vi "client.vi"() -> ()   [LabVIEW 2019]
uses:
  <vilib>/NI/STM/TCP/Read Meta Data (TCP Ref).vi
  <vilib>/NI/STM/TCP/Get Connection Reference (TCP).vi
  <vilib>/NI/STM/TCP/Read Meta Data (TCP Clst).vi
  <vilib>/NI/STM/TCP/Write Message (TCP).vi
  <vilib>/NI/STM/TCP/Read Message (TCP).vi
  <vilib>/NI/STM/NI STM.lvlib
panel:
  out "MOVE Command":T1
  out "error  out":errorcluster
  in  "stop":bool
  in  "Target IP Address":string="192.168.150.9"
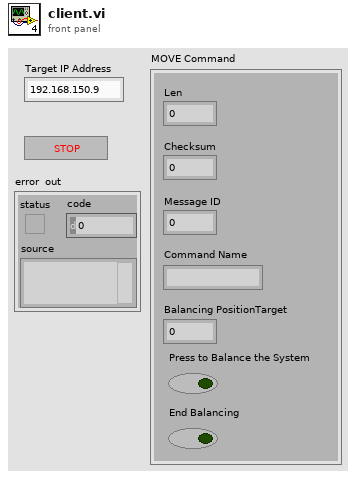
[diagram p1: front panel]
types:
  T1 = cluster{"Len":u8, "Checksum":u16, "Message ID":u16, "Command Name":string, "Balancing PositionTarget ":dbl, "Press to Balance the System":bool, "End Balancing":bool}
  T2 = typedef "NI STM.lvlib/TCP Connection Info.ctl" = cluster{"connection ID":refnum<k5>, "meta data":T3[]}
  T3 = typedef "NI STM.lvlib/MetaDataElement.ctl" = string
  T4 = cluster{"Len":u8, "Checksum":u16, "Message ID":u16, "Command Name":u32, "Balancing PositionTarget ":dbl, "Press to Balance the System":bool, "End Balancing":bool}
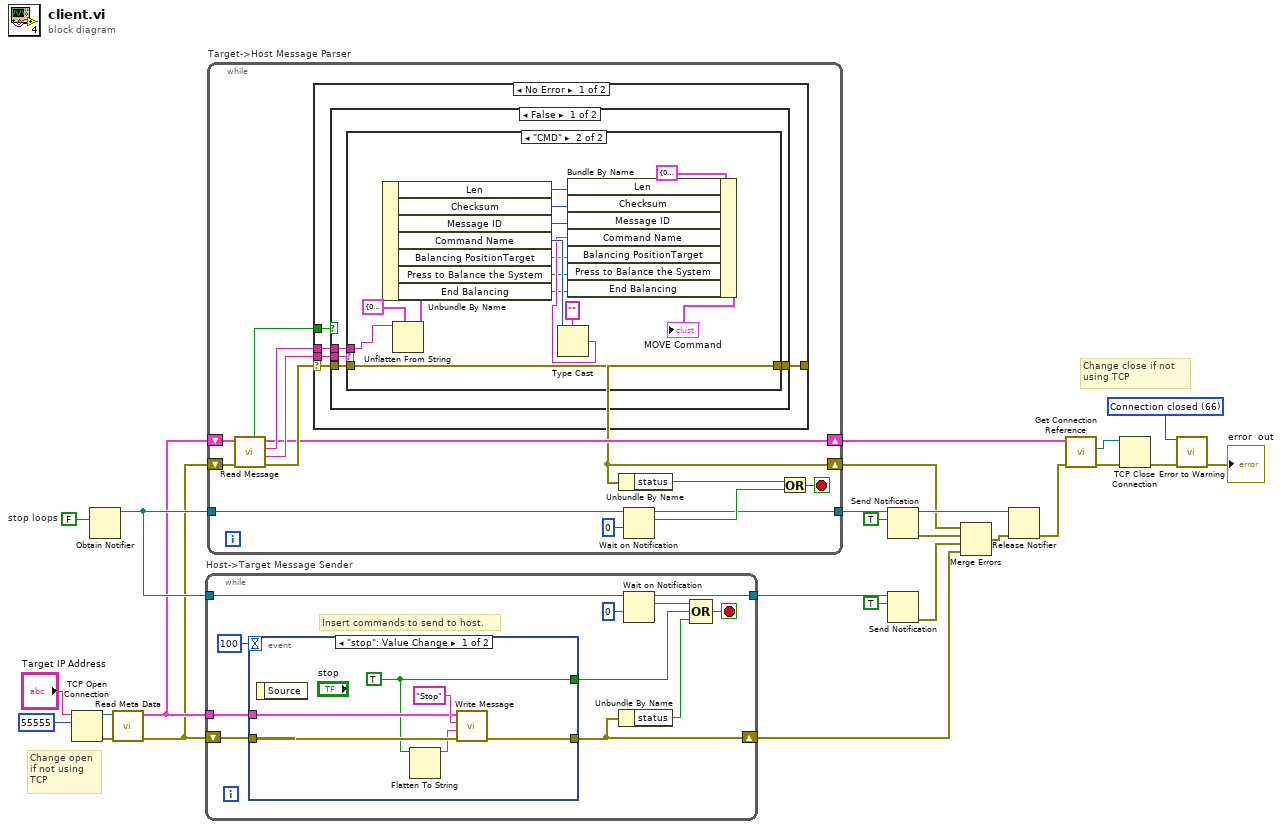
[diagram p0: block diagram]
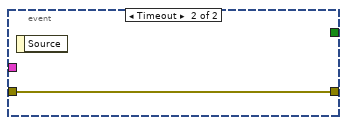
[diagram p2: hidden frame]
diagram:
  w11 = FALSE  # stop loops
  w23 = 66 items=["No Error", "Argument Error", "Memory Full", "Out of Zone", "End of File", "File Already Open", "Generic File IO Error", "File Not Found", "File Permission Error", "Disk Full", "Duplicate Path", "Too Many Files Open", "Not Enabled", "Resource File Not Found", "Cannot Add Resource", "Resource Not Found", "Image Not Found", "Image Memory Error", "Pen Does Not Exist", "Config Bad Type", "Config Token Not Found", "Config Parse Error", "Config Memory Error", "Bad External Code Format", "Bad External Code Offset", "External Code Not Present", "Null Window", "Destroy Window Mixup", "Null Menu", "Print Aborted", "Bad Print Record", "Print Driver Error", "Windows Error During Print", "Memory Error During Print", "Print Dialog Error", "Generic Print Error", "Invalid Device Refnum", "Device Not Found", "Device Parameter Error", "Device Unit Error", "Can't Open Device", "Device Call Aborted", "Generic Error", "Cancelled By User", "Object ID Too Low", "Object ID Too High", "Object Not In Heap", "Unknown Heap", "Bad DefProc ID", "DefProc Not In Table", "Message Out Of Range", "Null Method", "Unknown Message", "Manager Call Not Supported", "Bad address", "Connection In progress", "Connection timed out", "Connection is already in progress", "Network attribute not supported", "Network error", "Address in use", "System out of memory", "Connection aborted", "Connection refused", "Connection is not connected", "Connection is already connected", "Connection closed", "Initialize error (interapplication manager)", "Bad occurrence", "Wait on unbound occurrence handler", "Occurrence queue overflow", "Bad path", "Semaphore not signaled", "Unrecognized type (interapplication manager)"] ("1st Error to Convert")
  # "Change close if not using TCP"
  # "Change open if not using TCP"
  n1 = TCP Open Connection(address="Target IP Address", remote port or service name=u16 55555 ("remote port")) -> (connection ID=w7:refnum<k5>, error out=w6:errorcluster)  [unwired: 1 in, 2 out]
  n2 = Obtain Notifier(notification data type=w11) -> (notifier out=w14:refnum<notifier>)  [unwired: 3 in, 2 out]
  n3 = call-poly <vilib>:"Read Meta Data.vi"("error in"=w6, "connection ID"=w7) -> ("error out"=w8:errorcluster, "connection info out"=w9:T2)  [unwired: 1 in, 7 out]
  n4 = while "Host->Target Message Sender" {
    shift-right: [w28] -> w17
    shift-left: w8 -> [w36]
    tunnel: w9 -> [w35]
    tunnel: w14 -> [w32]
    tunnel: [w29] -> w15
    stop <- w30 stop-if-true
    # "Insert commands to send to host."
    n5 = event shown="[0] \"stop\": Value Change" {
      selector: _ -> [_ _]
      dyn-events: _ -> [_ _]
      timeout: 100 -> [_ _]
      tunnel: w35 -> [w41 _]
      tunnel: w36 -> [w40 w43]
      tunnel: [w38 _] -> w27
      tunnel: [w37 w43] -> w28
      event "stop": Value Change {
        w38 = TRUE ("stop")
        n6 = event-data() -> ()  [unwired: 2 out]
        n7 = Flatten To String(anything=w38) -> (data string=w39:string)  [unwired: 2 in, 3 out]
        n8 = call-poly <vilib>:"Write Message.vi"("error in"=w40, "data"=w39, "name"="Stop" ("Name"), "connection info in"=w41) -> ("error out"=w37:errorcluster)  [unwired: 1 in, 6 out]
      }
      event Timeout {
        n9 = event-data() -> ()  [unwired: 2 out]
      }
    }
    n10 = Unbundle By Name(w28) -> ("status"=w26:bool)
    n11 = Wait on Notification(notifier=w32, timeout in ms (-1)=0) -> (notifier out=w29:refnum<notifier>, notification=w34:bool)  [unwired: 2 in, 2 out]
    n12 = Compound Arithmetic op=OR(w34, w27, w26) -> (w30:bool)
  }
  n13 = while "Target->Host Message Parser" {
    shift-right: [w44] -> w3
    shift-left: w8 -> [w56]
    tunnel: w14 -> [w50]
    tunnel: [w46] -> w12
    shift-right: [w51] -> w10
    shift-left: w9 -> [w57]
    stop <- w47 stop-if-true
    n14 = call-poly <vilib>:"Read Message.vi"("error in"=w56, "connection info in"=w57) -> ("error out"=w52:errorcluster, "name"=w55:T3, "data string"=w54:string, "connection info out"=w51:T2, "timed out?"=w53:bool)  [unwired: 3 in, 2 out]
    n15 = case shown="No Error" w52 {
      selector: w52 -> [w59 w84]
      tunnel: w55 -> [w62 _]
      tunnel: w54 -> [w61 _]
      tunnel: w53 -> [w60 _]
      tunnel: [w58 w84] -> w44
      frame No Error {
        n16 = case shown="False" w60 {
          tunnel: w62 -> [w63 _]
          tunnel: w61 -> [w66 _]
          tunnel: w59 -> [w65 w83]
          tunnel: [w64 w83] -> w58
          frame False {
            n17 = case shown="\"CMD\"" w63 {
              tunnel: w66 -> [_ w81]
              tunnel: w65 -> [w67 w82]
              tunnel: [w67 w82] -> w64
              frame Default {
                # "Insert commands received from host."
              }
              frame "CMD" {
                n18 = Unflatten From String(type=T4 {"Len"=0, "Checksum"=0, "Message ID"=0, "Command Name"=0, "Balancing PositionTarget "=0.0, "Press to Balance the System"=FALSE, "End Balancing"=FALSE} ("MOVE Command 2"), binary string=w81) -> (value=w77:T4)  [unwired: 3 in, 2 out]
                n19 = Unbundle By Name(w77) -> ("Len"=w74:u8, "Checksum"=w73:u16, "Message ID"=w72:u16, "Command Name"=w79:u32, "Balancing PositionTarget"=w71:dbl, "Press to Balance the System"=w70:bool, "End Balancing"=w69:bool)
                n20 = Type Cast(type="", x=w79) -> (*(type *) &x=w75:string)
                n21 = Bundle By Name(cluster=T1 {"Len"=0, "Checksum"=0, "Message ID"=0, "Command Name"="", "Balancing PositionTarget "=0.0, "Press to Balance the System"=FALSE, "End Balancing"=FALSE} ("MOVE Command 2"), "Len"=w74, "Checksum"=w73, "Message ID"=w72, "Command Name"=w75, "Balancing PositionTarget"=w71, "Press to Balance the System"=w70, "End Balancing"=w69) -> (→"MOVE Command":T1)
              }
            }
          }
          frame True {
          }
        }
      }
      frame Error {
      }
    }
    n22 = Unbundle By Name(w44) -> ("status"=w45:bool)
    n23 = Wait on Notification(notifier=w50, timeout in ms (-1)=0) -> (notifier out=w46:refnum<notifier>, notification=w48:bool)  [unwired: 2 in, 2 out]
    n24 = Or(x=w45, y=w48) -> (x .or. y?=w47:bool)
  }
  n25 = Send Notification(notification=TRUE, notifier=w12) -> (notifier out=w20:refnum<notifier>, error out=w19:errorcluster)  [unwired: 1 in]
  n26 = Send Notification(notification=TRUE, notifier=w15) -> (error out=w18:errorcluster)  [unwired: 1 in, 1 out]
  n27 = Merge Errors(w3, w19, w18, w17) -> (w21:errorcluster)
  n28 = Release Notifier(notifier=w20, error in (no error)=w21) -> (error out=w22:errorcluster)  [unwired: 1 in, 2 out]
  n29 = call-poly <vilib>:"Get Connection Reference.vi"("error in"=w22, "connection info in"=w10) -> ("error out"=w2:errorcluster, "connection ID out"=w1:refnum<k5>)  [unwired: 8 out]
  n30 = TCP Close Connection(connection ID=w1, error in (no error)=w2) -> (error out=w24:errorcluster)  [unwired: 2 out]
  n31 = call <vilib>:"Error to Warning.vi"("1st Error to Convert"=w23, "error in"=w24) -> ("warning out"=→"error  out":errorcluster)  [unwired: 3 in, 10 out]
